vi "FPGA_Main.vi"() -> ()   [LabVIEW 2018]
uses:
  <vilib>/rvi/Emulation/niFpgaGetClockAttributes.vi
  <vilib>/rvi/Emulation/niFpgaSctlEmulationGetInTimedLoop.vi
  <vilib>/rvi/Emulation/niFpgaEmulationReportErrorSimple.vi
  <vilib>/rvi/eio/common/nirviEmuTemplateMethod_errors.vi
  <vilib>/rvi/interface/RandomDataEmulation/niFpgaRandomDataHandleErrors.vi
  <vilib>/rvi/Emulation/niFpgaCriticalErrorInLSC.vi
  <vilib>/rvi/Emulation/niFpgaProcessEmulError.vi
  <vilib>/eio/EIONode/EIONode.xnode
  <vilib>/rvi/DataTransferAndStorage/Container/XNode/niFpgaContainer.xnode
  <vilib>/rvi/interface/RandomDataEmulation/nirviRandomDataFpgaReadWriteTemplate.vi
panel:
  out "laser_AO Indicator":sgl format="%.5f"
  in  "frame_clock_timing":T1={"Frequency (periods/tick)"=0.0, "Phase offset (periods)"=0.0, "Scale factor"=0.999969482421875, "Amplitude offset"=0.0, "duty cycle (periods)"=0.5}
  in  "ephys_clock_timing":T1={"Frequency (periods/tick)"=0.0, "Phase offset (periods)"=0.0, "Scale factor"=0.999969482421875, "Amplitude offset"=0.0, "duty cycle (periods)"=0.5}
  in  "laser_trig__OFF Time":i16=2 caption="dio.trial_on_trig__ON Time"
  in  "laser_ctrl":bool
  in  "laser_trig__ON Time":i16=2 caption="dio.trial_on_trig__ON Time"
  out "Loop Rate for clock loop":u32
  in  "left_texture_ctrl":bool
  in  "right_texture_ctrl":bool
  in  "whisker_video_ctrl":bool
  in  "trial_ephys_ctrl":bool
  out "ephys_clock_DO":bool
  out "trial_on_ctrl_DO":bool
  out "trial_iti_ctrl_DO":bool
  out "trial_ephys_ctrl_DO":bool
  out "right_texture_ctrl_DO":bool
  out "left_texture_ctrl_DO":bool
  out "water_valve_ctrl_DO":bool
  out "lick_signal_DI":bool
  out "whisker_video_ctrl_DO":bool
  out "frame_clock_DO":bool
  out "aClck_DI":bool
  in  "laser_AO":sgl format="%.5f"
  in  "AO2":sgl format="%.5f"
  in  "right_wall_AO":sgl format="%.5f"
  in  "left_wall_AO":sgl format="%.5f"
  in  "water_valve_ctrl":bool
  in  "water_valve_ctrl_ON Time":i16=2 caption="dio.trial_on_trig__ON Time"
  out "Loop Rate for Inputs and Outputs Loop":u32
  out "Vy1":sgl format="%_4g"
  out "Vx1":sgl format="%_4g"
  out "Vy0":sgl format="%_4g"
  out "Vx0":sgl format="%_4g"
  out "Loop Rate for Digital Trigger Loop":u32
  out "Iteration":u64
  # "usec"
  # "usec"
  # "usec"
  # "Vdc"
  # "Vdc"
  # "Vdc"
  # "Vdc"
  # "ON Time(ms)"
  # "OFF Time(ms)"
  # "laser"
  # "msec"
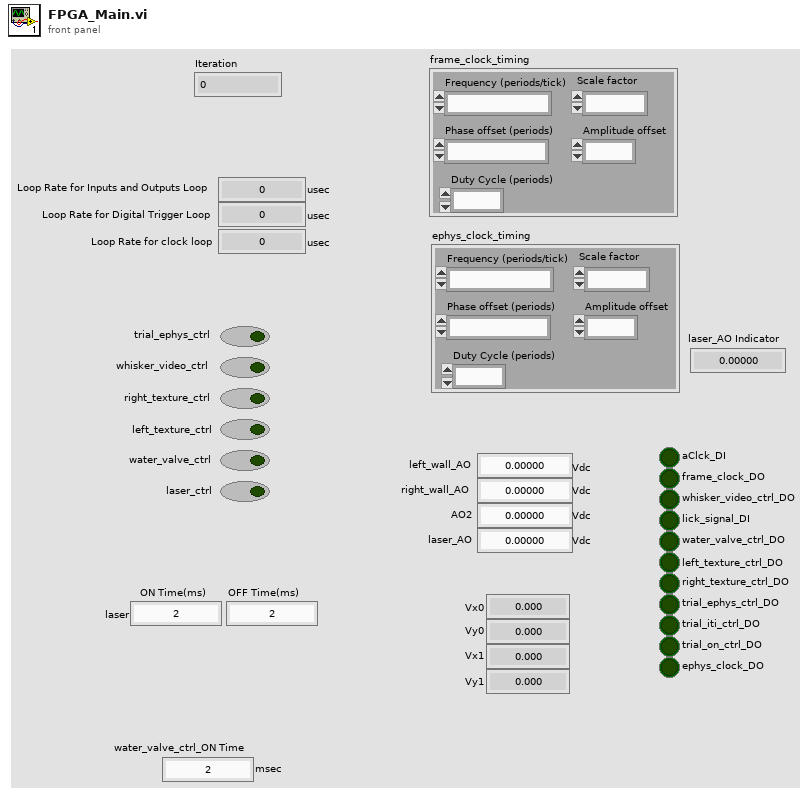
[diagram p1: front panel]
types:
  T1 = cluster{"Frequency (periods/tick)":fxp<+,32,0>, "Phase offset (periods)":fxp<+,32,0>, "Scale factor":fxp<+/-,16,1>, "Amplitude offset":fxp<+/-,16,16>, "duty cycle (periods)":fxp<+,32,0>}
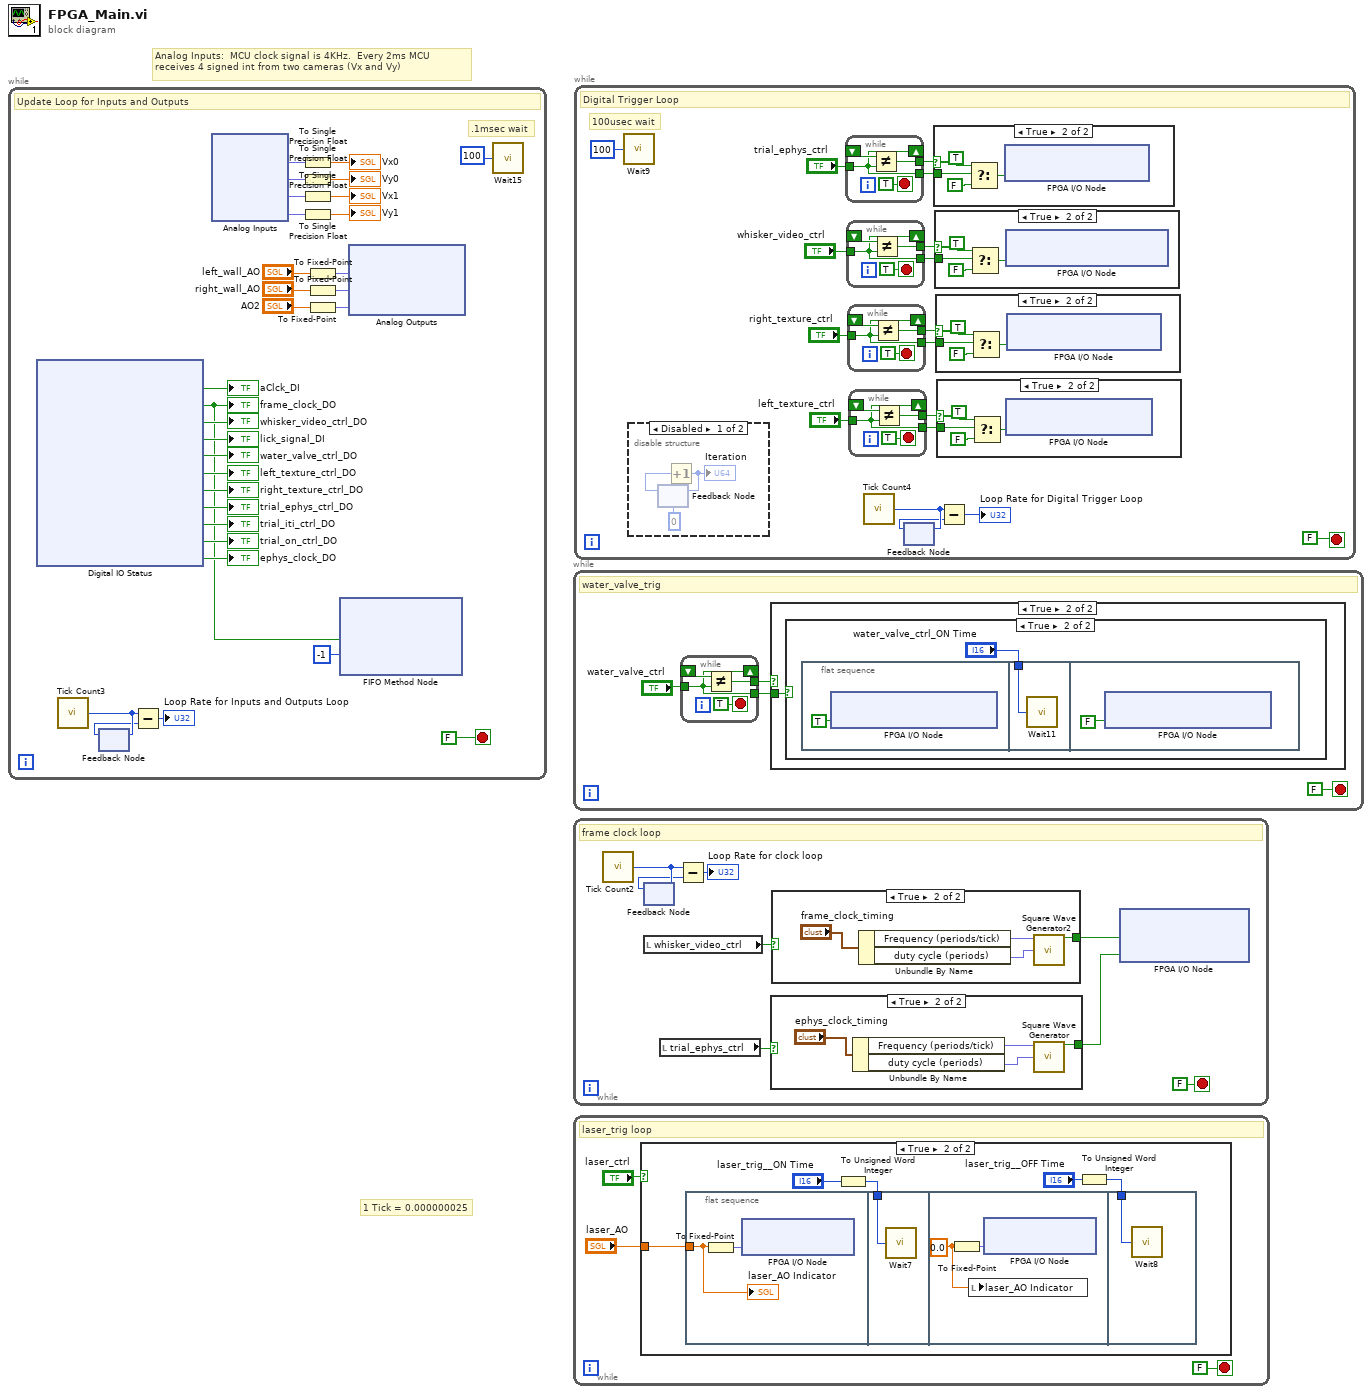
[diagram p0: block diagram]
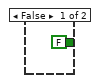
[diagram p2: hidden frame]
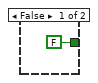
[diagram p3: hidden frame]
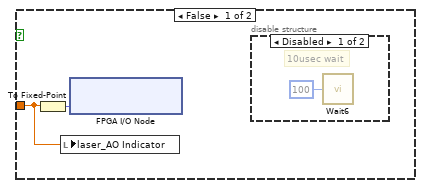
[diagram p4: hidden frame]
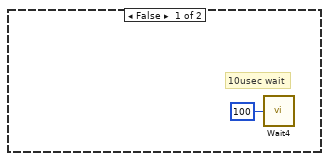
[diagram p6: hidden frame]
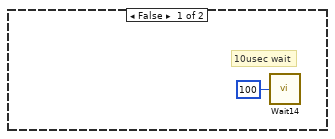
[diagram p7: hidden frame]
diagram:
  # "Analog Inputs:  MCU clock signal is 4KHz.  Every 2ms MCU receives 4 signed int from two cameras (Vx and Vy)"
  # "1 Tick = 0.000000025"
  n1 = while {
    stop <- FALSE stop-if-true
    # ".1msec wait"
    # "Update Loop for Inputs and Outputs"
    n2 = xnode "Digital IO Status"() -> ("aClck_DI"=→"aClck_DI":bool, "frame_clock_DO"=w1:bool, "whisker_video_trig_DO"=→"whisker_video_ctrl_DO":bool, "lick_signal_DO"=→"lick_signal_DI":bool, "water_valve_trigger_DO"=→"water_valve_ctrl_DO":bool, "left_texture_trig_DO"=→"left_texture_ctrl_DO":bool, "right_texture_trig_DO"=→"right_texture_ctrl_DO":bool, "trial_ephys_trig_DO"=→"trial_ephys_ctrl_DO":bool, "trial_iti_trig_DO"=→"trial_iti_ctrl_DO":bool, "trial_on_trig_DO"=→"trial_on_ctrl_DO":bool, "ephys_clock_DO"=→"ephys_clock_DO":bool)  [unwired: 11 in, 11 out]
    "frame_clock_DO" <- w1
    n3 = call "Tick Count3"() -> ("Tick Count(uSec)"=w29:u32)
    n4 = feedback #1() -> (w28:u32)  [unwired: 1 in]
    n5 = feedback-in #1(w29) -> ()
    n6 = Subtract(x=w29, y=w28) -> (x-y=→"Loop Rate for Inputs and Outputs Loop":u32)
    n7 = xnode "Analog Inputs"() -> ("Vx0"=w26:fxp<+/-,26,5>, "Vy0"=w25:fxp<+/-,26,5>, "Vx1"=w24:fxp<+/-,26,5>, "Vy1"=w23:fxp<+/-,26,5>)  [unwired: 4 in, 4 out]
    n8 = To Single Precision Float(number=w26) -> (single precision float=→"Vx0":sgl)
    n9 = To Single Precision Float(number=w25) -> (single precision float=→"Vy0":sgl)
    n10 = To Single Precision Float(number=w24) -> (single precision float=→"Vx1":sgl)
    n11 = To Single Precision Float(number=w23) -> (single precision float=→"Vy1":sgl)
    n12 = To Fixed-Point(number="left_wall_AO") -> (fixed-point=w13:fxp<+/-,32,16>)  [unwired: 1 in]
    n13 = To Fixed-Point(number="right_wall_AO") -> (fixed-point=w14:fxp<+/-,32,16>)  [unwired: 1 in]
    n14 = To Fixed-Point(number="AO2") -> (fixed-point=w15:fxp<+/-,32,16>)  [unwired: 1 in]
    n15 = xnode ("FIFO Method Node")("Element"=w1, "Timeout"=-1) -> ()  [unwired: 1 in, 2 out]
    n16 = xnode "Analog Outputs"("left_wall_AO"=w13, "right_wall_AO"=w14, "Mod2/AO2"=w15) -> ()  [unwired: 3 in, 3 out]
    n17 = call "Wait15"("Count(uSec)"=u32 100 ("Count(mSec)")) -> ()  [unwired: 1 out]
  }
  n18 = while {
    stop <- FALSE stop-if-true
    # "water_valve_trig"
    n19 = while {
      shift-right: [w43] -> _
      shift-left: _ -> [w45]
      tunnel: "water_valve_ctrl" -> [w43]
      tunnel: [w44] -> w33
      tunnel: [w43] -> w32
      stop <- TRUE stop-if-true
      n20 = Not Equal?(x=w45, y=w43) -> (x != y?=w44:bool)
    }
    n21 = case shown="True" w33 {
      tunnel: w32 -> [_ w37]
      frame False {
        # "10usec wait"
        n22 = call "Wait4"("Count(uSec)"=u32 100 ("Count(mSec)")) -> ()  [unwired: 1 out]
      }
      frame True {
        n23 = case shown="True" w37 {
          frame False {
            # "10usec wait"
            n24 = call "Wait14"("Count(uSec)"=u32 100 ("Count(mSec)")) -> ()  [unwired: 1 out]
          }
          frame True {
            n25 = flat-sequence {
              tunnel: "water_valve_ctrl_ON Time" -> [w41]
              frame #0 {
                n26 = xnode "FPGA I/O Node"("water_valve_trigger_DO"=TRUE ("frame_clock_DO")) -> ()  [unwired: 1 in, 1 out]
              }
              frame #1 {
                n27 = call "Wait11"("Count(mSec)"=w41) -> ()  [unwired: 1 out]
              }
              frame #2 {
                n28 = xnode "FPGA I/O Node"("water_valve_trigger_DO"=FALSE ("frame_clock_DO")) -> ()  [unwired: 1 in, 1 out]
              }
            }
          }
        }
      }
    }
  }
  n29 = while {
    stop <- FALSE stop-if-true
    # "frame clock loop"
    n30 = call "Tick Count2"() -> ("Tick Count(uSec)"=w53:u32)
    n31 = feedback #2() -> (w52:u32)  [unwired: 1 in]
    n32 = feedback-in #2(w53) -> ()
    n33 = local read "whisker_video_ctrl"() -> (w49:bool)
    n34 = local read "trial_ephys_ctrl"() -> (w48:bool)
    n35 = Subtract(x=w53, y=w52) -> (x-y=→"Loop Rate for clock loop":u32)
    n36 = case shown="True" w48 {
      tunnel: [FALSE ("square wave out") w56] -> w47
      frame False {
      }
      frame True {
        n37 = Unbundle By Name("ephys_clock_timing") -> ("Frequency (periods/tick)"=w58:fxp<+,32,0>, "duty cycle (periods)"=w57:fxp<+,32,0>)
        n38 = call "Square Wave Generator"("frequency (periods/tick)"=w58, "duty cycle (periods)"=w57) -> ("square wave out"=w56:bool)  [unwired: 13 in]
      }
    }
    n39 = case shown="True" w49 {
      tunnel: [FALSE ("square wave out") w61] -> w50
      frame False {
      }
      frame True {
        n40 = Unbundle By Name("frame_clock_timing") -> ("Frequency (periods/tick)"=w63:fxp<+,32,0>, "duty cycle (periods)"=w62:fxp<+,32,0>)
        n41 = call "Square Wave Generator2"("frequency (periods/tick)"=w63, "duty cycle (periods)"=w62) -> ("square wave out"=w61:bool)  [unwired: 13 in]
      }
    }
    n42 = xnode "FPGA I/O Node"("frame_clock_DO"=w50, "ephys_clock_DO"=w47) -> ()  [unwired: 2 in, 2 out]
  }
  n43 = while {
    stop <- FALSE stop-if-true
    # "laser_trig loop"
    n44 = case shown="True" "laser_ctrl" {
      tunnel: "laser_AO" -> [w68 w75]
      frame False {
        n45 = To Fixed-Point(number=w68) -> (fixed-point=w69:fxp<+/-,32,16>)  [unwired: 1 in]
        n46 = local write "laser_AO Indicator"(w68) -> ()
        n47 = xnode ("FPGA I/O Node")("laser_trig_AO"=w69) -> ()  [unwired: 1 in, 1 out]
        n48 = disable-structure shown="Disabled" {
          frame Disabled {
            # "10usec wait"
            n49 = call "Wait6"("Count(uSec)"=u32 100 ("Count(mSec)")) -> ()  [unwired: 1 out]
          }
          frame Enabled {
          }
        }
      }
      frame True {
        n50 = flat-sequence {
          tunnel: w75 -> [w76]
          tunnel: w73 -> [w78]
          tunnel: w71 -> [w81]
          frame #0 {
            n51 = To Fixed-Point(number=w76) -> (fixed-point=w77:fxp<+/-,32,16>)  [unwired: 1 in]
            n52 = xnode ("FPGA I/O Node")("laser_trig_AO"=w77) -> ()  [unwired: 1 in, 1 out]
            "laser_AO Indicator" <- w76
          }
          frame #1 {
            n53 = call "Wait7"("Count(mSec)"=w78) -> ()  [unwired: 1 out]
          }
          frame #2 {
            w79 = sgl 0.0
            n54 = To Fixed-Point(number=w79) -> (fixed-point=w80:fxp<+/-,32,16>)  [unwired: 1 in]
            n55 = local write "laser_AO Indicator"(w79) -> ()
            n56 = xnode ("FPGA I/O Node")("laser_trig_AO"=w80) -> ()  [unwired: 1 in, 1 out]
          }
          frame #3 {
            n57 = call "Wait8"("Count(mSec)"=w81) -> ()  [unwired: 1 out]
          }
        }
        n58 = To Unsigned Word Integer(number="laser_trig__ON Time") -> (unsigned 16bit integer=w73:u16)
        n59 = To Unsigned Word Integer(number="laser_trig__OFF Time") -> (unsigned 16bit integer=w71:u16)
      }
    }
  }
  n60 = while {
    stop <- FALSE stop-if-true
    # "100usec wait"
    # "Digital Trigger Loop"
    n61 = call "Wait9"("Count(uSec)"=u32 100 ("Count(mSec)")) -> ()  [unwired: 1 out]
    n62 = disable-structure shown="Disabled" {
      frame Disabled {
        n63 = feedback #3(u64 0) -> (w109:u64)
        n64 = Increment(x=w109) -> (x+1=w108:u64)
        "Iteration" <- w108
        n65 = feedback-in #3(w108) -> ()
      }
      frame Enabled {
      }
    }
    n66 = while {
      shift-right: [w103] -> _
      shift-left: _ -> [w105]
      tunnel: "trial_ephys_ctrl" -> [w103]
      tunnel: [w104] -> w84
      tunnel: [w103] -> w85
      stop <- TRUE stop-if-true
      n67 = Not Equal?(x=w105, y=w103) -> (x != y?=w104:bool)
    }
    n68 = while {
      shift-right: [w130] -> _
      shift-left: _ -> [w132]
      tunnel: "whisker_video_ctrl" -> [w130]
      tunnel: [w131] -> w94
      tunnel: [w130] -> w93
      stop <- TRUE stop-if-true
      n69 = Not Equal?(x=w132, y=w130) -> (x != y?=w131:bool)
    }
    n70 = while {
      shift-right: [w122] -> _
      shift-left: _ -> [w124]
      tunnel: "right_texture_ctrl" -> [w122]
      tunnel: [w123] -> w90
      tunnel: [w122] -> w91
      stop <- TRUE stop-if-true
      n71 = Not Equal?(x=w124, y=w122) -> (x != y?=w123:bool)
    }
    n72 = while {
      shift-right: [w114] -> _
      shift-left: _ -> [w116]
      tunnel: "left_texture_ctrl" -> [w114]
      tunnel: [w115] -> w89
      tunnel: [w114] -> w88
      stop <- TRUE stop-if-true
      n73 = Not Equal?(x=w116, y=w114) -> (x != y?=w115:bool)
    }
    n74 = call "Tick Count4"() -> ("Tick Count(uSec)"=w98:u32)
    n75 = feedback #4() -> (w97:u32)  [unwired: 1 in]
    n76 = feedback-in #4(w98) -> ()
    n77 = case shown="True" w84 {
      tunnel: w85 -> [_ w102]
      frame False {
      }
      frame True {
        n78 = Select(t=TRUE ("frame_clock_DO"), s=w102, f=FALSE ("frame_clock_DO")) -> (s? t:f=w99:bool)
        n79 = xnode "FPGA I/O Node"("trial_ephys_trig_DO"=w99) -> ()  [unwired: 1 in, 1 out]
      }
    }
    n80 = case shown="True" w94 {
      tunnel: w93 -> [_ w129]
      frame False {
      }
      frame True {
        n81 = Select(t=TRUE ("frame_clock_DO"), s=w129, f=FALSE ("frame_clock_DO")) -> (s? t:f=w126:bool)
        n82 = xnode "FPGA I/O Node"("whisker_video_trig_DO"=w126) -> ()  [unwired: 1 in, 1 out]
      }
    }
    n83 = case shown="True" w90 {
      tunnel: w91 -> [_ w121]
      frame False {
      }
      frame True {
        n84 = Select(t=TRUE ("frame_clock_DO"), s=w121, f=FALSE ("frame_clock_DO")) -> (s? t:f=w118:bool)
        n85 = xnode "FPGA I/O Node"("right_texture_trig_DO"=w118) -> ()  [unwired: 1 in, 1 out]
      }
    }
    n86 = case shown="True" w89 {
      tunnel: w88 -> [_ w113]
      frame False {
      }
      frame True {
        n87 = Select(t=TRUE ("frame_clock_DO"), s=w113, f=FALSE ("frame_clock_DO")) -> (s? t:f=w110:bool)
        n88 = xnode "FPGA I/O Node"("left_texture_trig_DO"=w110) -> ()  [unwired: 1 in, 1 out]
      }
    }
    n89 = Subtract(x=w98, y=w97) -> (x-y=→"Loop Rate for Digital Trigger Loop":u32)
  }
